vi "Write VI Interpreter.vi"(5 "VI Interpreter":refnum<class "VI Interpreter.lvclass">, 9 "PythonConverter_GUI in":refnum<class "PythonConverter_GUI.lvclass">) -> (3 "PythonConverter_GUI out":refnum<class "PythonConverter_GUI.lvclass">)   [LabVIEW 2014, in "Raspberry Pi Compatible Compiler for LabVIEW.lvlib" / "PythonConverter_GUI.lvclass"]
uses:
  PythonConverter_GUI.lvclass
  VI Interpreter/Classes/VI Interpreter/VI Interpreter.lvclass
  PythonConverter_GUI.lvclass/PythonConverter_GUI.ctl
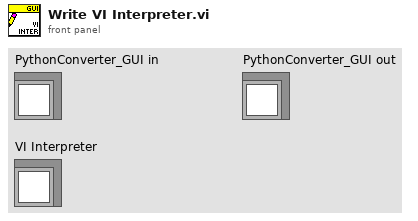
[diagram p1: front panel]
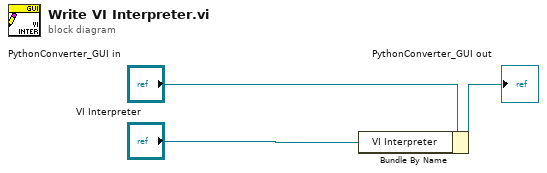
[diagram p0: block diagram]
diagram:
  n1 = Bundle By Name(cluster="PythonConverter_GUI in", "VI Interpreter"="VI Interpreter") -> (→"PythonConverter_GUI out":refnum<class "PythonConverter_GUI.lvclass">)
